vi "save B scan data.vi"(10 "Channel array in":dbl[][](array[numeric]), 11 "Scan save path":path) -> (3 "Size":i32[](array[numeric]))   [LabVIEW 2014]
uses:
  <vilib>/Utility/file.llb/Write To Spreadsheet File (DBL).vi
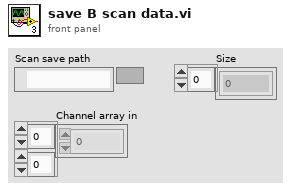
[diagram p1: front panel]
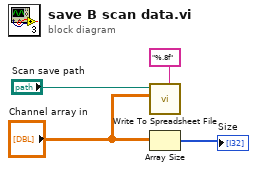
[diagram p0: block diagram]
diagram:
  n1 = call-poly <vilib>:"Write To Spreadsheet File.vi"("format (%.3f)"="%.8f", "2D data"="Channel array in", "file path (dialog if empty)"="Scan save path") -> ()  [unwired: 5 in, 1 out]
  n2 = Array Size(array="Channel array in") -> (size(s)=→"Size":i32[])
